vi "Init.vi"(0 "VISA resource name":refnum<visa-resource-name>, 5 "error in":errorcluster) -> (14 "SR865":T1, 19 "error out":errorcluster)   [LabVIEW 2018]
uses:
  SR865.ctl
  <vilib>/Instr/_visa.llb/VISA Open Access Mode.ctl
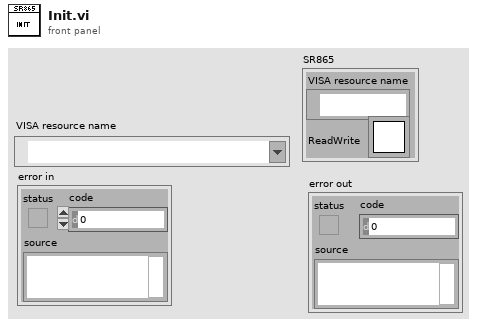
[diagram p1: front panel]
types:
  T1 = typedef "SR865.ctl" = cluster{"VISA resource name":refnum<visa-resource-name>, "ReadWrite":T2}
  T2 = typedef "Semaphore RefNum" = refnum<k1>
  T3 = typedef "VISA Open Access Mode.ctl" = u32
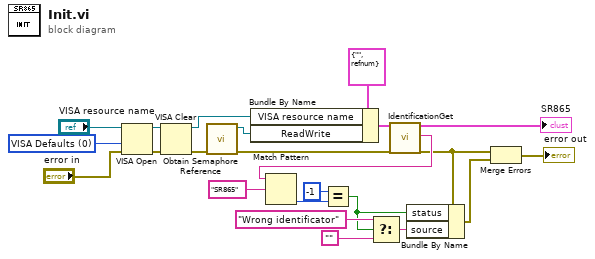
[diagram p0: block diagram]
diagram:
  w23 = T3 0 items=["VISA Defaults"=0, "Exclusive Lock"=1, "Load Configured Settings"=4] ("Access Mode")
  n1 = VISA Open(access mode=w23, error in (no error)="error in", VISA resource name="VISA resource name") -> (VISA resource name=w20:refnum<visa-resource-name>, error out=w19:errorcluster)  [unwired: 2 in]
  n2 = VISA Clear(VISA resource name=w20, error in (no error)=w19) -> (VISA resource name out=w3:refnum<visa-resource-name>, error out=w18:errorcluster)
  n3 = call <vilib>:"Obtain Semaphore Reference.vi"("error in (no error)"=w18) -> ("error out"=w12:errorcluster, "semaphore"=w2:T2)  [unwired: 4 in, 1 out]
  n4 = Bundle By Name(cluster=T1 {"VISA resource name"="", "ReadWrite"=refnum} ("SR865"), "VISA resource name"=w3, "ReadWrite"=w2) -> (w1:T1)
  n5 = call "IdentificationGet.vi"("SR865 in"=w1, "error in"=w12) -> ("SR865 out"=→"SR865":T1, "Identification"=w10:string, "error out"=w7:errorcluster)  [unwired: 15 in]
  n6 = Match Pattern(string=w10, regular expression="SR865") -> (offset past match=w6:i32)  [unwired: 1 in, 3 out]
  n7 = Equal?(x=-1 ("y"), y=w6) -> (x = y?=w14:bool)
  n8 = Select(t="Wrong identificator" ("source"), s=w14, f="") -> (s? t:f=w16:string)
  n9 = Bundle By Name(cluster=w7, "status"=w14, "source"=w16) -> (w9:errorcluster)
  n10 = Merge Errors(w7, w9) -> (→"error out":errorcluster)
